vi "Analyze.vi"(8 "error in (no error)":errorcluster, 10 "Image in":T1, 11 "Analyze SecondMomentum in":refnum<class "Analyze SecondMomentum.lvclass">) -> (0 "error out":errorcluster, 1 "Result":refnum<class "Analyze Results Base.lvclass">, 2 "Image out":T1, 3 "Analyze SecondMomentum out":refnum<class "Analyze SecondMomentum.lvclass">)   [LabVIEW 2020, in "Analyze.lvlib" / "Analyze SecondMomentum.lvclass"]
uses:
  Analyze SecondMomentum.lvclass
  C:/POLARIS Programme/POLARIS-AS-3-Cams/Submodules/HIJ Vision/Analyze/Analyze Classes/Analyze BaseClass/Analyze BaseClass/Analyze BaseClass.lvclass
  <vilib>/vision/Image Controls.llb/IMAQ Image.ctl
  Results and Overlays/Results Base/Analyze Results Base.lvclass
  Results and Overlays/Results Second Momentum/Analyze Results Second Momentum.lvclass
  C:/POLARIS Programme/POLARIS-AS-3-Cams/Submodules/HIJ Vision/Analyze/Results and Overlays/Results Base/Analyze Results Base.lvclass
  Results and Overlays/Results Second Momentum/Analyze Results Second Momentum.lvclass/Analyze Results Second Momentum.ctl
  Results and Overlays/Results Second Momentum/Write 1st M x 1.vi
  Results and Overlays/Results Second Momentum/Write 1st M y 1.vi
  Results and Overlays/Results Second Momentum/Write 2nd M x 1.vi
  Results and Overlays/Results Second Momentum/Write 2nd M y 1.vi
  Results and Overlays/Results Second Momentum/Write D x 1.vi
  Results and Overlays/Results Second Momentum/Write D y 1.vi
  Analyze BaseClass/Analyze BaseClass/Analyze BaseClass.lvclass
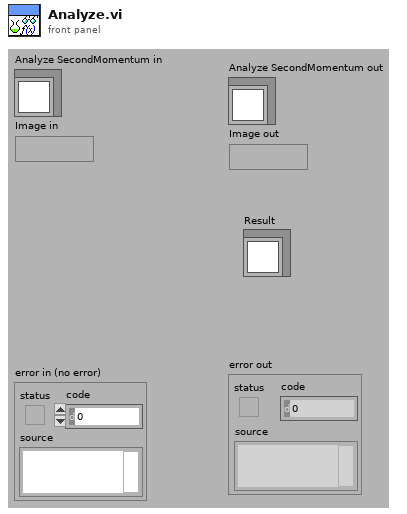
[diagram p1: front panel]
types:
  T1 = typedef "IMAQ Image.ctl" = refnum<image>
  T2 = typedef "ROI Descriptor" = cluster{"Global Rectangle":i32[], "Contours":cluster{"ID":enum32{"External", "Internal"}, "Type":u32, "Coordinates":i32[]}[]}
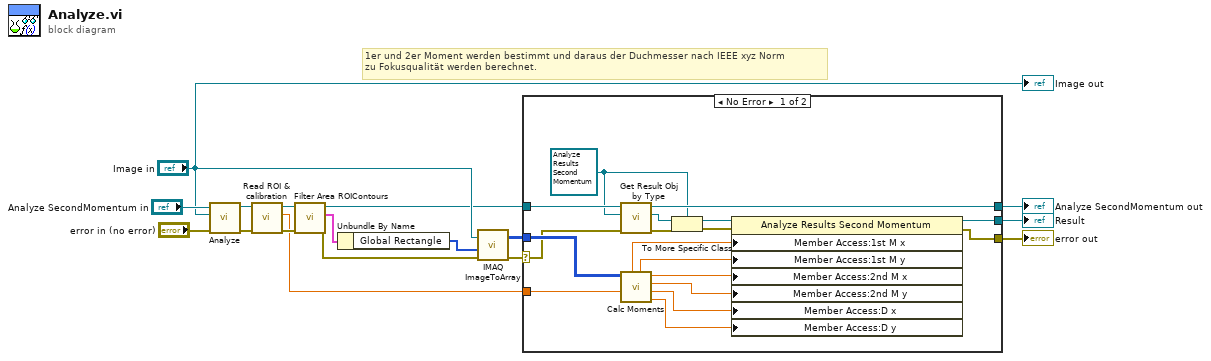
[diagram p0: block diagram]
diagram:
  # "1er und 2er Moment werden bestimmt und daraus der Duchmesser nach IEEE xyz Norm\nzu Fokusqualität werden berechnet."
  n1 = call-parent "Analyze.vi"("error in (no error)"="error in (no error)", "Image in"="Image in", "Analyze BaseClass in"="Analyze SecondMomentum in") -> ("error out"=w7:errorcluster, "Analyze BaseClass out"=w6:refnum<class "Analyze SecondMomentum.lvclass">)  [unwired: 5 in, 2 out]
  n2 = call-dynamic "Read ROI & calibration.vi"("error in (no error)"=w7, "Analyze BaseClass in"=w6) -> ("error out"=w17:errorcluster, "calibration mm/px"=w14:dbl[unit], "Analyze BaseClass out"=w16:refnum<class "Analyze SecondMomentum.lvclass">)  [unwired: 6 in, 1 out]
  n3 = call-dynamic "Filter Area ROIContours.vi"("error in (no error)"=w17, "Analyze BaseClass in"=w16) -> ("error out"=w13:errorcluster, "ROI of Area type"=w12:T2, "Analyze BaseClass out"=w2:refnum<class "Analyze SecondMomentum.lvclass">)  [unwired: 7 in]
  n4 = Unbundle By Name(w12) -> ("Global Rectangle"=w11:i32[])
  n5 = call "IMAQ ImageToArray"("error in (no error)"=w13, "Optional Rectangle"=w11, "Image"="Image in") -> ("error out"=w4:errorcluster, "Image Pixels (I16)"=w10:i16[][])  [unwired: 1 in, 3 out]
  n6 = case shown="No Error" w4 {
    selector: w4 -> [w20 w37]
    tunnel: [w26 w37] -> w15
    tunnel: w14 -> [w28 _]
    tunnel: w10 -> [w35 _]
    tunnel: [w27 _] -> w5
    tunnel: w2 -> [w25 w36]
    tunnel: [w24 w36] -> w1
    frame No Error {
      w21 = refnum<class "Analyze Results Second Momentum.lvclass"> refnum ("Analyze Results Second Momentum.lvclass")
      n7 = call "Get Result Obj by Type.vi"("error in (no error)"=w20, "Parameter Type"=w21, "Analyze BaseClass in"=w25) -> ("error out"=w23:errorcluster, "Parameter"=w22:refnum<class "Analyze Results Base.lvclass">, "Analyze BaseClass out"=w24:refnum<class "Analyze SecondMomentum.lvclass">)  [unwired: 5 in, 1 out]
      n8 = call "Calc Moments.vi"("Calibration"=w28, "image array"=w35) -> ("Durchmesser Y"=w29:dbl[unit], "Durchmesser X"=w30:dbl[unit], "2nd Moment y"=w31:dbl[unit], "2nd Moment x"=w32:dbl[unit], "1st Moment y"=w33:dbl[unit], "1st Moment x"=w34:dbl[unit])  [unwired: 4 in]
      n9 = To More Specific Class(target class=w21, reference=w22, error in=w23) -> (specific class reference=w18:refnum<class "Analyze Results Second Momentum.lvclass">, error out=w19:errorcluster)
      n10 = property class="Analyze Results Second Momentum"(reference=w18, error in=w19, "Member Access:1st M x"=w34, "Member Access:1st M y"=w33, "Member Access:2nd M x"=w32, "Member Access:2nd M y"=w31, "Member Access:D x"=w30, "Member Access:D y"=w29) -> (reference out=w27:refnum<class "Analyze Results Second Momentum.lvclass">, error out=w26:errorcluster)
    }
    frame Error {
    }
  }
  "error out" <- w15
  "Analyze SecondMomentum out" <- w1
  "Result" <- w5
  "Image out" <- "Image in"
